vi "deleteFromIndices.vi"(9 "indices to delete":i32[](array[numeric]), 11 "vector":dbl[](array[numeric])) -> (2 "vector restricted":dbl[](array[numeric]))   [LabVIEW 2017]
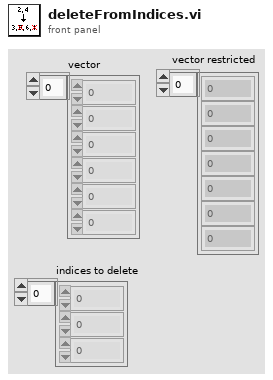
[diagram p1: front panel]
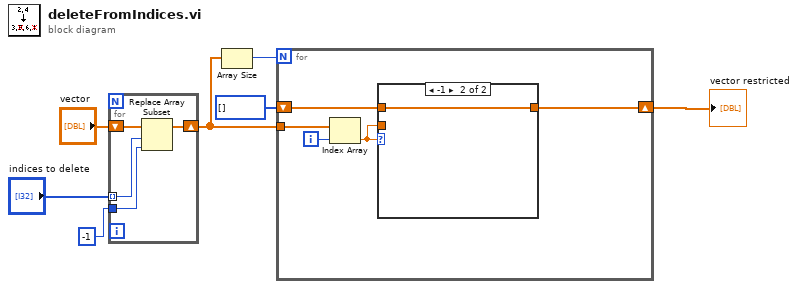
[diagram p0: block diagram]
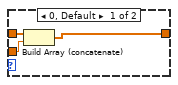
[diagram p2: hidden frame]
diagram:
  n1 = for {
    shift-right: [w9] -> w2
    shift-left: "vector" -> [w11]
    tunnel: "indices to delete" -> [w10] mode=indexing
    tunnel: -1 -> [w8]
    n2 = Replace Array Subset(array=w11, new element=w8, index=w10) -> (w9:dbl[])
  }
  n3 = Array Size(array=w2) -> (size(s)=w1:i32)
  n4 = for {
    N: w1 -> [_]
    tunnel: w2 -> [w16]
    shift-right: [w12] -> w3
    shift-left: i32[] [] ("Array 3") -> [w13]
    i -> [w15]
    n5 = Index Array(array=w16, index=w15) -> (element=w14:dbl)
    n6 = case shown="-1" w14 {
      tunnel: w14 -> [w19 _]
      tunnel: w13 -> [w18 w20]
      tunnel: [w17 w20] -> w12
      frame 0, Default {
        n7 = Build Array (concatenate)(w18, w19) -> (w17:dbl[])
      }
      frame -1 {
      }
    }
  }
  "vector restricted" <- w3
